vi "accelerometer_real_test.vi"(0 "Speed Index":i32, 1 "x,y,z?":i32=1, 2 "i":i32, 3 "speed subarray":dbl[](array[numeric]), 4 "transposed array":dbl[][](array[numeric])) -> (5 "Acceleration":dbl, 6 "Speed":dbl)   [LabVIEW 2025]
uses:
  468687ae-6b61-4150-b139-1e5540973179.vi
panel:
  # "Data from: https://data.mendeley.com/datasets/5rrxw7y5bj/1"
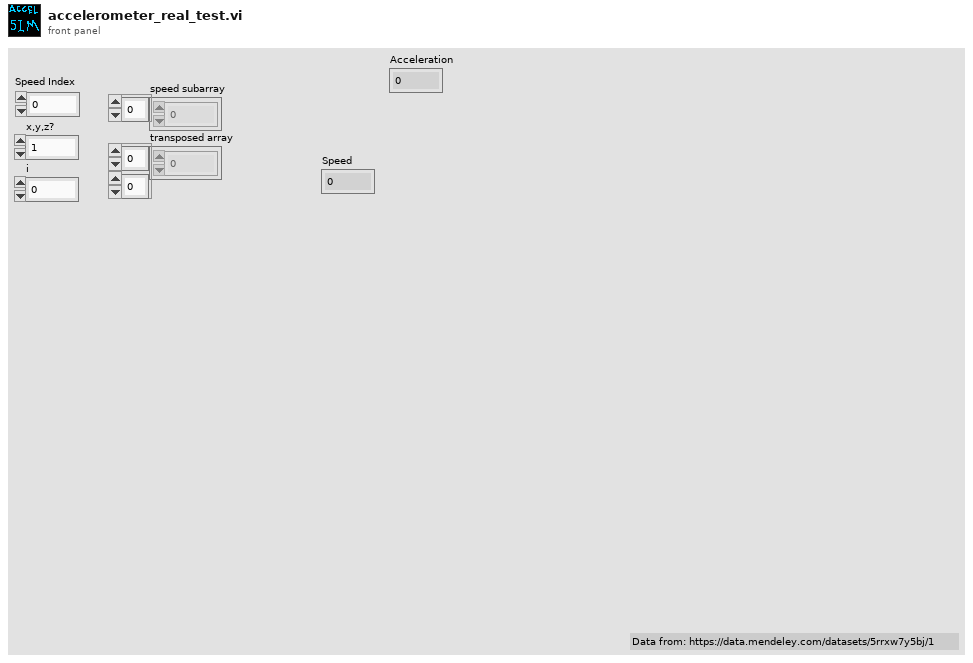
[diagram p1: front panel]
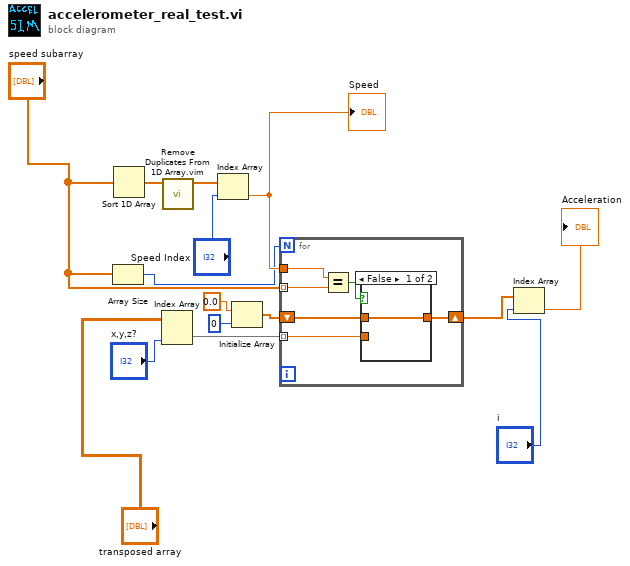
[diagram p0: block diagram]
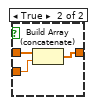
[diagram p2: hidden frame]
diagram:
  n1 = Array Size(array="speed subarray") -> (size(s)=w11:i32)
  n2 = Sort 1D Array(array="speed subarray") -> (sorted array=w8:dbl[])
  n3 = Index Array(array="transposed array", index (col)="x,y,z?") -> (element=w15:dbl[])  [unwired: 1 in]
  n4 = call "Remove Duplicates From 1D Array.vim"("array"=w8) -> ("array with duplicates removed"=w10:dbl[])  [unwired: 10 in]
  n5 = Index Array(array=w10, index="Speed Index") -> (element=w12:dbl)
  "Speed" <- w12
  n6 = Initialize Array(0.0 ("element"), 0 ("dimension size")) -> (w13:dbl[])
  n7 = for {
    N: w11 -> [_]
    tunnel: "speed subarray" -> [w18] mode=indexing
    tunnel: w12 -> [w21]
    shift-right: [w16] -> w5
    shift-left: w13 -> [w19]
    tunnel: w15 -> [w17] mode=indexing
    n8 = Equal?(x=w21, y=w18) -> (x = y?=w20:bool)
    n9 = case shown="False" w20 {
      tunnel: w19 -> [w22 w25]
      tunnel: [w22 w24] -> w16
      tunnel: w17 -> [_ w23]
      frame False {
      }
      frame True {
        n10 = Build Array (concatenate)(w25, w23) -> (w24:dbl[])
      }
    }
  }
  n11 = Index Array(array=w5, index="i") -> (element=→"Acceleration":dbl)
